vi "ADI_IMU_ADIS16448_ReadRegister.vi"(8 "error in (no error)":errorcluster, 10 "ADIS16448 Register":T1=86 items=["SEQ_CNT"=58, "SMPL_PRD"=54, "SENS_AVG"=56, "MSC_CTRL"=52, "ERROR_FLAGS"=60, "TEMP"=44, "BARO"=40, "Z_MAG"=36, "Y_MAG"=32, "X_MAG"=28, "Z_ACCEL"=24, "Y_ACCEL"=20, "X_ACCEL"=16, "Z_GYRO"=12, "Y_GYRO"=8, "X_GYRO"=4, "PID"=86], 11 "SPIDevRef in":T2) -> (0 "error out":errorcluster, 2 "Register Value":u16, 3 "SPIDevRef out":T2)   [LabVIEW 2016, in "ADIS16448_IMU.lvlib"]
uses:
  ADIS16448_IMU.lvlib
  <vilib>/Rock Robotics/WPI/SPI/WPI_SPIDevRef.ctl
  <vilib>/Rock Robotics/SystemInterfaces/spilib/spi_bus.ctl
  ADI_IMU_ADIS16448_Registers.ctl
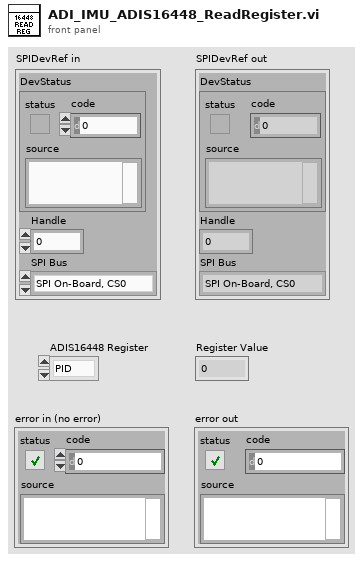
[diagram p1: front panel]
types:
  T1 = typedef "ADIS16448_IMU.lvlib/ADI_IMU_ADIS16448_Registers.ctl" = u8
  T2 = typedef "WPI_SPIDevRef.ctl" = cluster{"DevStatus":errorcluster, "Handle":i32, "SPI Bus":T3}
  T3 = typedef "spi_bus.ctl" = enum16{"SPI On-Board, CS0", "SPI On-Board, CS1", "SPI On-Board, CS2", "SPI On-Board, CS3", "SPI MXP", "Invalid"}
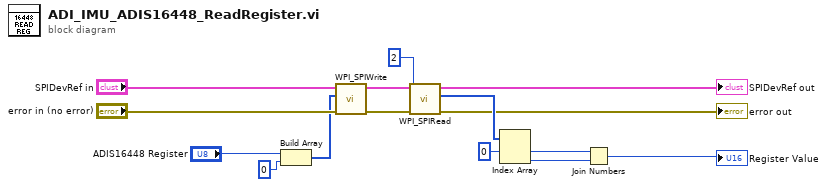
[diagram p0: block diagram]
diagram:
  n1 = Build Array("ADIS16448 Register", u8 0 ("element")) -> (w8:T1[])
  n2 = call <vilib>:"WPI_SPIWrite.vi"("error in (no error)"="error in (no error)", "Data To Send"=w8, "SPIDevRef"="SPIDevRef in") -> ("error out"=w3:errorcluster, "SPIDevRef"=w4:T2)  [unwired: 7 out]
  n3 = call <vilib>:"WPI_SPIRead.vi"("error in (no error)"=w3, "Num to Read"=2, "SPIDevRef"=w4) -> ("error out"=→"error out":errorcluster, "Received Data"=w10:u8[], "SPIDevRef"=→"SPIDevRef out":T2)  [unwired: 6 in]
  n4 = Index Array(array=w10, index #1=0 ("index")) -> (element #1=w7:u8, element #2=w6:u8)  [unwired: 1 in]
  n5 = Join Numbers(hi=w7, lo=w6) -> ((hi.lo)=→"Register Value":u16)
